vi "PCO_GetCameraBusyStatus.vi"(8 "error in (no error)":errorcluster {"code" format="%x"}, 11 "ph":u64) -> (0 "error out":errorcluster {"code" format="%x"}, 1 "wCameraBusyState":u16(ring) items=["not busy", "busy"], 2 "ErrorMessage":i32 format="%x", 3 "ph out":u64)   [LabVIEW 2020, in "SDK.lvlib" / "TimingControl.lvlib"]
doc: "<b>Description:</b>\nThis function returns the current busy status of the camera. The busy status is according to the <busy> hardware signal at the camera output and can be checked before a PCO_ForceTrigger command to ensure that this command does start a new exposure. Due to response and processing times caused by the interface and / or the operating system, the delay between the delivered status and the current status may be several milliseconds. For exact synchronization to external events the hardware signal <busy> must be used.\n\n<b>Supported camera type:</b>\npco.edge, pco.1600, pco.2000, pco.4000\n\n<b>Descriptor dependency:</b>\nNone"
uses:
  TimingControl.lvlib
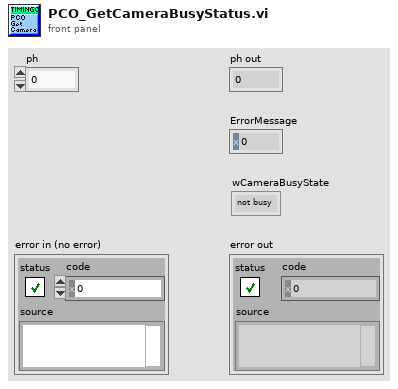
[diagram p1: front panel]
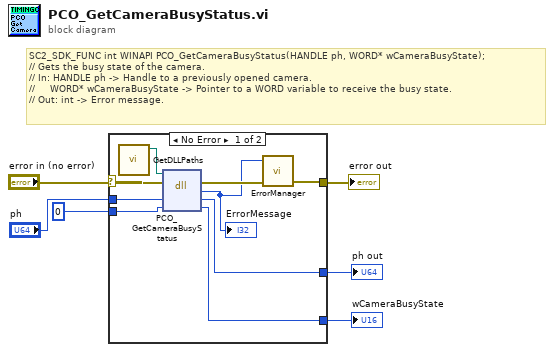
[diagram p0: block diagram]
diagram:
  # "SC2_SDK_FUNC int WINAPI PCO_GetCameraBusyStatus(HANDLE ph, WORD* wCameraBusyState);\n// Gets the busy state of the camera.\n// In: HANDLE ph -> Handle to a previously opened camera.\n//     WORD* wCameraBusyState -> Pointer to a WORD variable to receive the busy state.\n// Out: int -> Error message."
  n1 = case shown="No Error" "error in (no error)" {
    selector: "error in (no error)" -> [w11 w18]
    tunnel: "ph" -> [w15 w17]
    tunnel: [w14 w17] -> w5
    tunnel: u16 0 ("wCameraBusyState") -> [w13 w16]
    tunnel: [w12 w16] -> w3
    tunnel: [w9 w18] -> w2
    frame No Error {
      n2 = call "GetDLLPaths.vi"() -> ("SC2_Cam_Path"=w7:path)  [unwired: 9 in, 2 out]
      n3 = dll-call lib="?" fn="PCO_GetCameraBusyStatus"(path in=w7, error in=w11, "ph"=w15, "wCameraBusyState"=w13) -> (error out=w10:errorcluster, "return type"=w8:i32, "ph"=w14:u64, "wCameraBusyState"=w12:u16)  [unwired: 1 in, 1 out]
      "ErrorMessage" <- w8
      n4 = call "ErrorManager.vi"("error in (no error)"=w10, "error code"=w8) -> ("error out"=w9:errorcluster)  [unwired: 3 in]
    }
    frame Error {
    }
  }
  "ph out" <- w5
  "wCameraBusyState" <- w3
  "error out" <- w2
